vi "Config File Checker.vi"(8 "Error In":errorcluster) -> (0 "error out":errorcluster, 1 "Password":string, 2 "output cluster":T1={"LH"={"Go Up"={"Min Speed"=120.0, "Max Speed"=10.0, "Min Time"=1.82, "Max Time"=3.7, "Min Run Current"=0.0, "Max Run Current"=10.0, "Min Stall Current"=0.0, "Max Stall Current"=25.0, "Min Stall Force"=170.0, "Max Stall Force"=320.0, "Min Stroke"=170.0, "Max Stroke"=320.0}, "Go Down"={"Min Speed"=10.0, "Max Speed"=250.0, "Min Travel Time"=1.82, "Max Travel Time"=3.7, "Min Run Current"=0.0, "Max Run Current"=10.0}, "Shipping"={"Min Distance"=150.0, "Max Distance"=300.0, "Setpoint"=5.0}, "Anti-Pinch"={"Min Force"=5.0, "Max Force"=15.0}}, "RH"={"Go Up"={"Min Speed"=120.0, "Max Speed"=10.0, "Min Time"=1.82, "Max Time"=3.7, "Min Run Current"=0.0, "Max Run Current"=10.0, "Min Stall Current"=0.0, "Max Stall Current"=25.0, "Min Stall Force"=170.0, "Max Stall Force"=320.0, "Min Stroke"=170.0, "Max Stroke"=320.0}, "Go Down"={"Min Speed"=10.0, "Max Speed"=250.0, "Min Travel Time"=1.82, "Max Travel Time"=3.7, "Min Run Current"=0.0, "Max Run Current"=10.0}, "Shipping"={"Min Distance"=150.0, "Max Distance"=300.0, "Setpoint"=5.0}, "Anti-Pinch"={"Min Force"=5.0, "Max Force"=15.0}}, "W 601 FR RH Std"={"Go Up"={"Min Speed"=10.0, "Max Speed"=250.0, "Min Time"=0.5, "Max Time"=4.3, "Min Run Current"=0.0, "Max Run Current"=10.0, "Min Stall Current"=0.0, "Max Stall Current"=25.0, "Min Stall Force"=170.0, "Max Stall Force"=320.0, "Min Stroke"=254.4, "Max Stroke"=270.4}, "Go Down"={"Min Speed"=10.0, "Max Speed"=250.0, "Min Travel Time"=0.5, "Max Travel Time"=4.3, "Min Run Current"=0.0, "Max Run Current"=10.0}, "Shipping"={"Min Distance"=5.0, "Max Distance"=15.0, "Setpoint"=5.0}, "Anti-Pinch"={"Min Force"=5.0, "Max Force"=15.0}}, "W 601 FR LH Std"={"Go Up"={"Min Speed"=10.0, "Max Speed"=250.0, "Min Time"=0.5, "Max Time"=4.3, "Min Run Current"=0.0, "Max Run Current"=10.0, "Min Stall Current"=0.0, "Max Stall Current"=25.0, "Min Stall Force"=170.0, "Max Stall Force"=320.0, "Min Stroke"=254.4, "Max Stroke"=270.4}, "Go Down"={"Min Speed"=10.0, "Max Speed"=250.0, "Min Travel Time"=0.5, "Max Travel Time"=4.3, "Min Run Current"=0.0, "Max Run Current"=10.0}, "Shipping"={"Min Distance"=5.0, "Max Distance"=15.0, "Setpoint"=5.0}, "Anti-Pinch"={"Min Force"=5.0, "Max Force"=15.0}}, "W 601 RR RH Std"={"Go Up"={"Min Speed"=10.0, "Max Speed"=250.0, "Min Time"=0.5, "Max Time"=4.3, "Min Run Current"=0.0, "Max Run Current"=10.0, "Min Stall Current"=0.0, "Max Stall Current"=25.0, "Min Stall Force"=170.0, "Max Stall Force"=320.0, "Min Stroke"=254.4, "Max Stroke"=270.4}, "Go Down"={"Min Speed"=10.0, "Max Speed"=250.0, "Min Travel Time"=0.5, "Max Travel Time"=4.3, "Min Run Current"=0.0, "Max Run Current"=10.0}, "Shipping"={"Min Distance"=5.0, "Max Distance"=15.0, "Setpoint"=5.0}, "Anti-Pinch"={"Min Force"=5.0, "Max Force"=15.0}}, "W 601 RR LH Std"={"Go Up"={"Min Speed"=10.0, "Max Speed"=250.0, "Min Time"=0.5, "Max Time"=4.3, "Min Run Current"=0.0, "Max Run Current"=10.0, "Min Stall Current"=0.0, "Max Stall Current"=25.0, "Min Stall Force"=170.0, "Max Stall Force"=320.0, "Min Stroke"=254.4, "Max Stroke"=270.4}, "Go Down"={"Min Speed"=10.0, "Max Speed"=250.0, "Min Travel Time"=0.5, "Max Travel Time"=4.3, "Min Run Current"=0.0, "Max Run Current"=10.0}, "Shipping"={"Min Distance"=5.0, "Max Distance"=15.0, "Setpoint"=5.0}, "Anti-Pinch"={"Min Force"=5.0, "Max Force"=15.0}}, "W 601 FR RH AP"={"Go Up"={"Min Speed"=10.0, "Max Speed"=250.0, "Min Time"=0.5, "Max Time"=4.3, "Min Run Current"=0.0, "Max Run Current"=10.0, "Min Stall Current"=0.0, "Max Stall Current"=25.0, "Min Stall Force"=170.0, "Max Stall Force"=320.0, "Min Stroke"=254.4, "Max Stroke"=270.4}, "Go Down"={"Min Speed"=10.0, "Max Speed"=250.0, "Min Travel Time"=0.5, "Max Travel Time"=4.3, "Min Run Current"=0.0, "Max Run Current"=10.0}, "Shipping"={"Min Distance"=5.0, "Max Distance"=15.0, "Setpoint"=5.0}, "Anti-Pinch"={"Min Force"=5.0, "Max Force"=15.0}}, "W 601 FR LH AP"={"Go Up"={"Min Speed"=10.0, "Max Speed"=250.0, "Min Time"=0.5, "Max Time"=4.3, "Min Run Current"=0.0, "Max Run Current"=10.0, "Min Stall Current"=0.0, "Max Stall Current"=25.0, "Min Stall Force"=170.0, "Max Stall Force"=320.0, "Min Stroke"=254.4, "Max Stroke"=270.4}, "Go Down"={"Min Speed"=10.0, "Max Speed"=250.0, "Min Travel Time"=0.5, "Max Travel Time"=4.3, "Min Run Current"=0.0, "Max Run Current"=10.0}, "Shipping"={"Min Distance"=5.0, "Max Distance"=15.0, "Setpoint"=5.0}, "Anti-Pinch"={"Min Force"=5.0, "Max Force"=15.0}}, "W 601 RR RH AP"={"Go Up"={"Min Speed"=10.0, "Max Speed"=250.0, "Min Time"=0.5, "Max Time"=4.3, "Min Run Current"=0.0, "Max Run Current"=10.0, "Min Stall Current"=0.0, "Max Stall Current"=25.0, "Min Stall Force"=170.0, "Max Stall Force"=320.0, "Min Stroke"=254.4, "Max Stroke"=270.4}, "Go Down"={"Min Speed"=10.0, "Max Speed"=250.0, "Min Travel Time"=0.5, "Max Travel Time"=4.3, "Min Run Current"=0.0, "Max Run Current"=10.0}, "Shipping"={"Min Distance"=5.0, "Max Distance"=15.0, "Setpoint"=5.0}, "Anti-Pinch"={"Min Force"=5.0, "Max Force"=15.0}}, "W 601 RR LH AP"={"Go Up"={"Min Speed"=10.0, "Max Speed"=250.0, "Min Time"=0.5, "Max Time"=4.3, "Min Run Current"=0.0, "Max Run Current"=10.0, "Min Stall Current"=0.0, "Max Stall Current"=25.0, "Min Stall Force"=170.0, "Max Stall Force"=320.0, "Min Stroke"=254.4, "Max Stroke"=270.4}, "Go Down"={"Min Speed"=10.0, "Max Speed"=250.0, "Min Travel Time"=0.5, "Max Travel Time"=4.3, "Min Run Current"=0.0, "Max Run Current"=10.0}, "Shipping"={"Min Distance"=5.0, "Max Distance"=15.0, "Setpoint"=5.0}, "Anti-Pinch"={"Min Force"=5.0, "Max Force"=15.0}}}, 3 "Shipping":dbl)   [LabVIEW 2017]
doc: "V1.1:\n- changed the location of searching and creating the file"
uses:
  controls/All Specs.ctl
  controls/Specifications.ctl
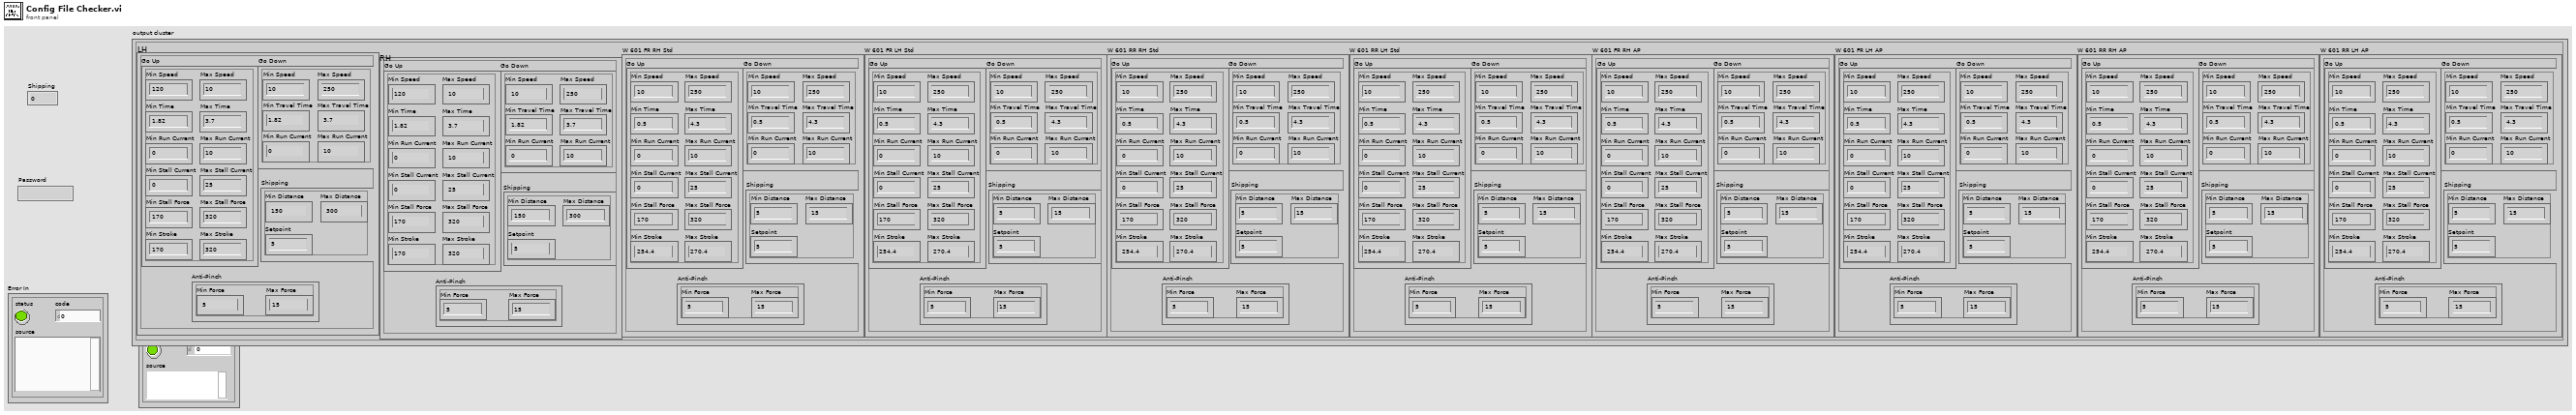
[diagram p1: front panel]
types:
  T1 = typedef "All Specs.ctl" = cluster{"LH":T2, "RH":T2, "W 601 FR RH Std":T2, "W 601 FR LH Std":T2, "W 601 RR RH Std":T2, "W 601 RR LH Std":T2, "W 601 FR RH AP":T2, "W 601 FR LH AP":T2, "W 601 RR RH AP":T2, "W 601 RR LH AP":T2}
  T2 = typedef "Specifications.ctl" = cluster{"Go Up":cluster{"Min Speed":dbl, "Max Speed":dbl, "Min Time":dbl, "Max Time":dbl, "Min Run Current":dbl, "Max Run Current":dbl, "Min Stall Current":dbl, "Max Stall Current":dbl, "Min Stall Force":dbl, "Max Stall Force":dbl, "Min Stroke":dbl, "Max Stroke":dbl}, "Go Down":cluster{"Min Speed":dbl, "Max Speed":dbl, "Min Travel Time":dbl, "Max Travel Time":dbl, "Min Run Current":dbl, "Max Run Current":dbl}, "Shipping":cluster{"Min Distance":dbl, "Max Distance":dbl, "Setpoint":dbl}, "Anti-Pinch":cluster{"Min Force":dbl, "Max Force":dbl}}
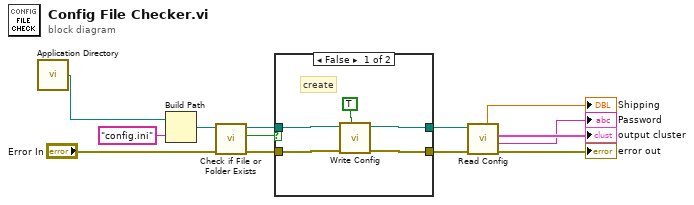
[diagram p0: block diagram]
diagram:
  n1 = call <vilib>:"Application Directory.vi"() -> ("Application Directory"=w1:path)
  n2 = Build Path(base path=w1, name or relative path="config.ini") -> (appended path=w11:path)
  n3 = call <vilib>:"Check if File or Folder Exists.vi"("error in (no error)"="Error In", "path"=w11) -> ("error out"=w8:errorcluster, "file or folder exists?"=w10:bool, "dup path"=w9:path)  [unwired: 7 in]
  n4 = case shown="False" w10 {
    tunnel: [w17 w20] -> w7
    tunnel: w9 -> [w18 w20]
    tunnel: w8 -> [w15 w19]
    tunnel: [w16 w19] -> w6
    frame False {
      # "create"
      n5 = call "Write Config.vi"("New File?"=TRUE, "error in (no error)"=w15, "file path"=w18) -> ("error out"=w16:errorcluster, "file path out"=w17:path)  [unwired: 7 in]
    }
    frame True {
    }
  }
  n6 = call "Read Config.vi"("error in"=w6, "file path"=w7) -> ("error out"=→"error out":errorcluster, "Password"=→"Password":string, "output cluster"=→"output cluster":T1, "Shipping"=→"Shipping":dbl)  [unwired: 5 in, 1 out]
